vi "GUI Write Sampling Status.vi"(7 "status label":string="stat3", 8 "error in":errorcluster, 10 "total samples":i64, 11 "data":T1) -> (0 "error out":errorcluster)   [LabVIEW 2020]
doc: "Updates status of sampling. Can generate error, but will exdcute even with input error."
uses:
  adc/ADC Data Packet.ctl
  varilib/SGUI Assign Multiple Strings With Tags By Label.vi
  varilib/varilib.lvlib
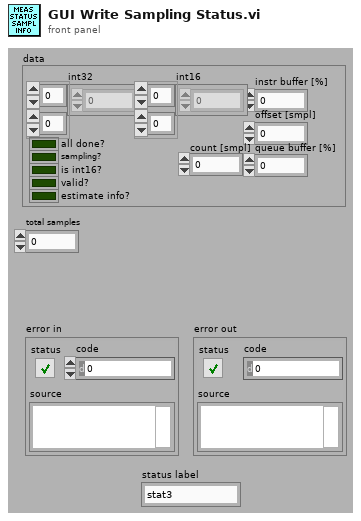
[diagram p1: front panel]
types:
  T1 = typedef "ADC Data Packet.ctl" = cluster{"int32":i32[][], "int16":i16[][], "offset [smpl]":i64, "count [smpl]":i32, "is int16?":bool, "all done?":bool, "sampling?":bool, "instr buffer [%]":dbl, "queue buffer [%]":dbl, "valid?":bool, "estimate info?":bool}
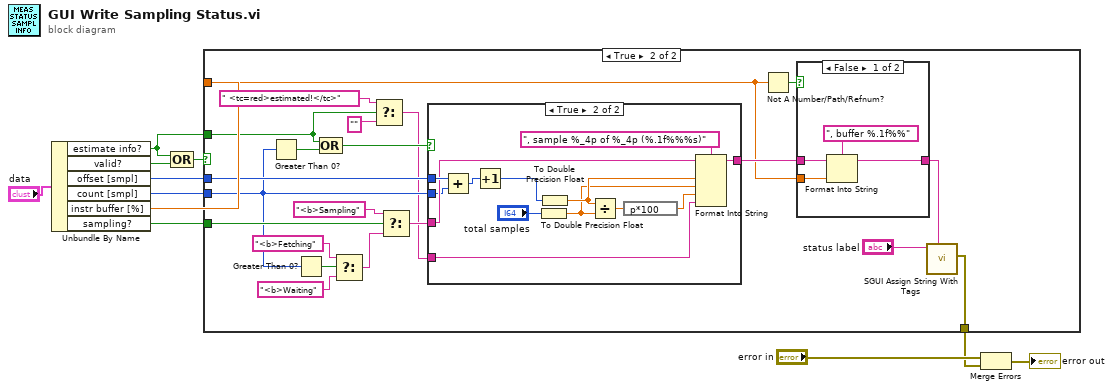
[diagram p0: block diagram]
diagram:
  n1 = Unbundle By Name("data") -> ("estimate info?"=w1:bool, "valid?"=w3:bool, "offset [smpl]"=w5:i64, "count [smpl]"=w6:i32, "instr buffer [%]"=w4:dbl, "sampling?"=w7:bool)
  n2 = Compound Arithmetic op=OR(w1, w3) -> (w2:bool)
  n3 = case shown="True" w2 {
    tunnel: [_ w29] -> w9
    tunnel: w7 -> [_ w28]
    tunnel: w6 -> [_ w20]
    tunnel: w5 -> [_ w22]
    tunnel: w4 -> [_ w13]
    tunnel: w1 -> [_ w17]
    frame False {
    }
    frame True {
      n4 = Greater Than 0?(x=w20) -> (x > 0?=w19:bool)
      n5 = Greater Than 0?(x=w20) -> (x > 0?=w25:bool)
      n6 = Compound Arithmetic op=OR(w17, w19) -> (w18:bool)
      n7 = Select(t="<b>Fetching" ("format string"), s=w25, f="<b>Waiting" ("format string")) -> (s? t:f=w26:string)
      n8 = Select(t=" <tc=red>estimated!</tc>" ("format string"), s=w17, f="" ("format string")) -> (s? t:f=w14:string)
      n9 = Select(t="<b>Sampling" ("format string"), s=w28, f=w26) -> (s? t:f=w21:string)
      n10 = case shown="True" w18 {
        tunnel: [w38 w50] -> w32
        tunnel: w22 -> [_ w49]
        tunnel: w21 -> [w38 w43]
        tunnel: w20 -> [_ w40]
        tunnel: w14 -> [_ w39]
        frame False {
        }
        frame True {
          n11 = Add(x=w49, y=w40) -> (x+y=w48:i64)
          n12 = Increment(x=w48) -> (x+1=w46:i64)
          n13 = To Double Precision Float(number="total samples") -> (double precision float=w41:dbl)
          n14 = To Double Precision Float(number=w46) -> (double precision float=w42:dbl)
          n15 = Divide(x=w42, y=w41) -> (x/y=w45:dbl)
          n16 = expression code="p*100"(w45) -> (w44:dbl)
          n17 = Format Into String(format string=", sample %_4p of %_4p (%.1f%%%s)", initial string=w43, w42, w41, w44, w39) -> (resulting string=w50:string)  [unwired: 1 in, 1 out]
        }
      }
      n18 = Not A Number/Path/Refnum?(number/path/refnum=w13) -> (NaN/Path/Refnum?=w12:bool)
      n19 = case shown="False" w12 {
        tunnel: w32 -> [w35 w37]
        tunnel: [w34 w37] -> w31
        tunnel: w13 -> [w33 _]
        frame False {
          n20 = Format Into String(format string=", buffer %.1f%%", initial string=w35, w33) -> (resulting string=w34:string)  [unwired: 1 in, 1 out]
        }
        frame True {
        }
      }
      n21 = call-poly "SGUI Assign String With Tags.vi"("label(s) (empty)"="status label", "string (empty)"=w31) -> ("error out"=w29:errorcluster)  [unwired: 8 in, 1 out]
    }
  }
  n22 = Merge Errors("error in", w9) -> (→"error out":errorcluster)
